vi "EnviaEmail.vi"(5 "subject":string, 6 "password":string, 7 "mensagem":string, 8 "SMTP":string, 9 "username":string, 10 "porta":string, 11 "Para":string[](array[string])) -> (2 "notificaoes rapidas-out":string)   [LabVIEW 2018]
uses:
  <vilib>/smtpClient/Set Message Text.vi
  <vilib>/smtpClient/LabVIEWSMTPClient.lvlib
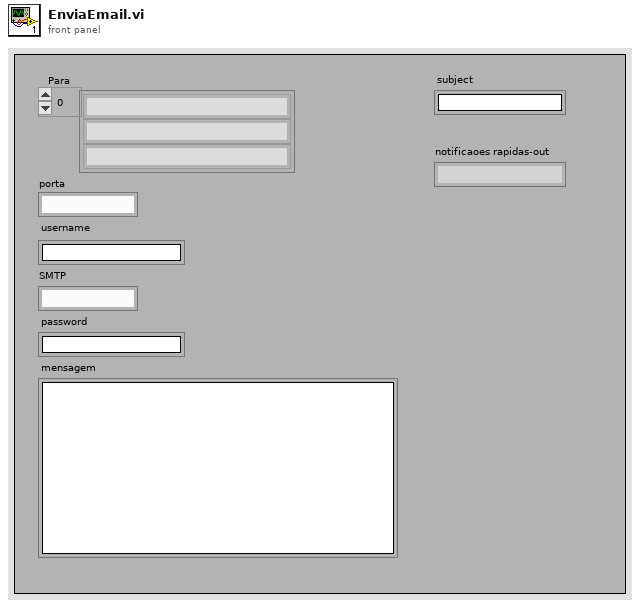
[diagram p1: front panel]
types:
  T1 = typedef "LabVIEWSMTPClient.lvlib/SmtpClientHandle.ctl" = refnum<k1>
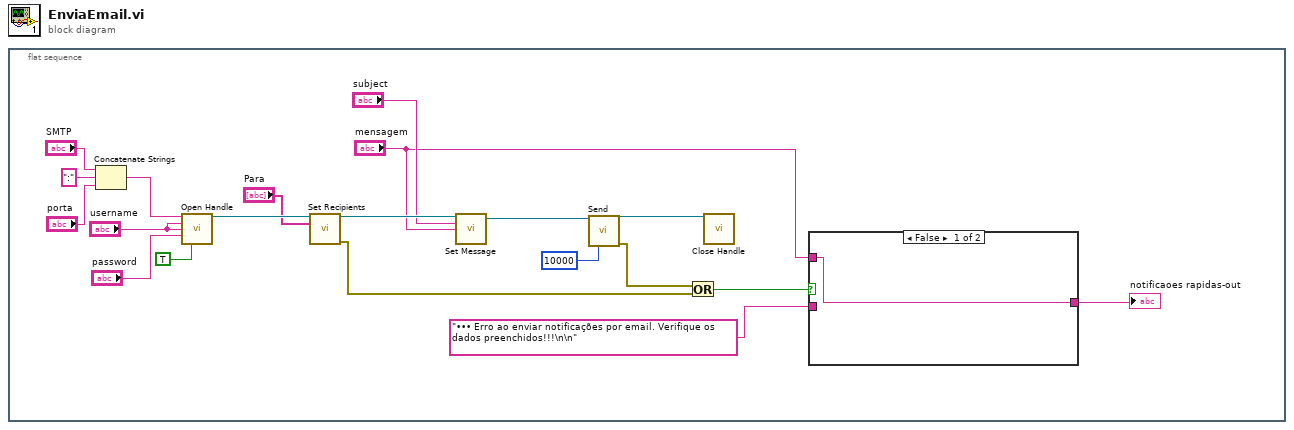
[diagram p0: block diagram]
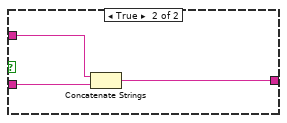
[diagram p2: hidden frame]
diagram:
  n1 = flat-sequence {
    frame #0 {
      n2 = Concatenate Strings("SMTP", ":" ("string"), "porta") -> (w14:string)
      n3 = call <vilib>:"Open Handle.vi"("server address"=w14, "from"="username", "username"="username", "password"="password", "use TLS (false)"=TRUE) -> ("handle out"=w17:T1)  [unwired: 9 in, 1 out]
      n4 = call <vilib>:"Set Recipients.vi"("handle in"=w17, "to"="Para") -> ("handle out"=w18:T1, "error out"=w5:errorcluster)  [unwired: 12 in]
      n5 = call-poly <vilib>:"Set Message.vi"("handle in"=w18, "subject"="subject", "plain text message"="mensagem") -> ("handle out"=w19:T1)  [unwired: 11 in, 1 out]
      n6 = call <vilib>:"Send.vi"("handle in"=w19, "timeout in ms (10000)"=10000) -> ("handle out"=w20:T1, "error out"=w6:errorcluster)  [unwired: 11 in, 1 out]
      n7 = Or(x=w6, y=w5) -> (x .or. y?=w4:bool)
      n8 = call <vilib>:"Close Handle.vi"("handle in"=w20) -> ()  [unwired: 13 in, 2 out]
      n9 = case shown="False" w4 {
        tunnel: "mensagem" -> [w21 w24]
        tunnel: "••• Erro ao enviar notificações por email. Verifique os dados preenchidos!!!\n\n" -> [_ w23]
        tunnel: [w21 w22] -> w1
        frame False {
        }
        frame True {
          n10 = Concatenate Strings(w24, w23) -> (w22:string)
        }
      }
      "notificaoes rapidas-out" <- w1
    }
  }
